vi "DAQStandarize.vi"(11 "Data in":waveform(dbl)[](array[waveform])) -> (3 "Data out":waveform(dbl)[](array[waveform]))   [LabVIEW 2019]
uses:
  Communication/TypeDef/#TypeDef_gForm.ctl
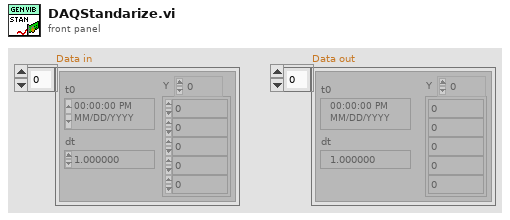
[diagram p1: front panel]
types:
  T1 = typedef "#TypeDef_gForm.ctl" = enum16{"1.5g", "6g"}
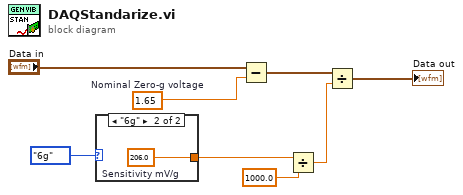
[diagram p0: block diagram]
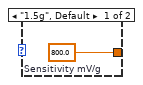
[diagram p2: hidden frame]
diagram:
  w3 = 1.65  # Nominal Zero-g voltage
  n1 = case shown="\"6g\"" #TypeDef_gForm."6g" ("G form") {
    tunnel: [w9 w10] -> w2
    frame "1.5g", Default {
      w9 = 800.0  # Sensitivity mV/g
    }
    frame "6g" {
      w10 = 206.0  # Sensitivity mV/g
    }
  }
  n2 = Subtract(x="Data in", y=w3) -> (x-y=w6:waveform(dbl)[])
  n3 = Divide(x=w2, y=1000.0) -> (x/y=w7:dbl)
  n4 = Divide(x=w6, y=w7) -> (x/y=→"Data out":waveform(dbl)[])
